vi "FieldAngleCalculation.vi"(8 "Previous Field Angle (rad)":sgl, 9 "Flux density magnitude (T)":sgl, 11 "Omega (rad/s)":sgl) -> (1 "New Field Angle (rad)":sgl, 2 "Bv (T)":sgl, 3 "Bu (T)":sgl)   [LabVIEW 2017]
uses:
  <vilib>/rvi/FXPMathLib/FxpSinAndCos/subVIs/nifxpmath_SinAndCos_SimConfig.ctl
  <vilib>/rvi/FXPMathLib/FxpSinAndCos/simVIs/DllFxpSinAndCosTemp_sub.vi
  <vilib>/rvi/FXPMathLib/FxpSinAndCos/XNode/nifxpmath_SinAndCos.xnode
panel:
  in  "Time Step (ms)":sgl=2.0
  # "Control parameters"
  # "Output"
  # "Inputs"
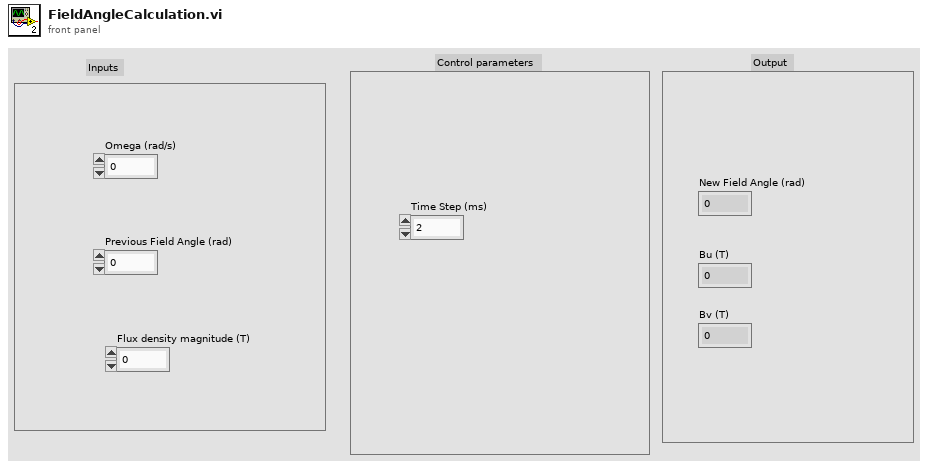
[diagram p1: front panel]
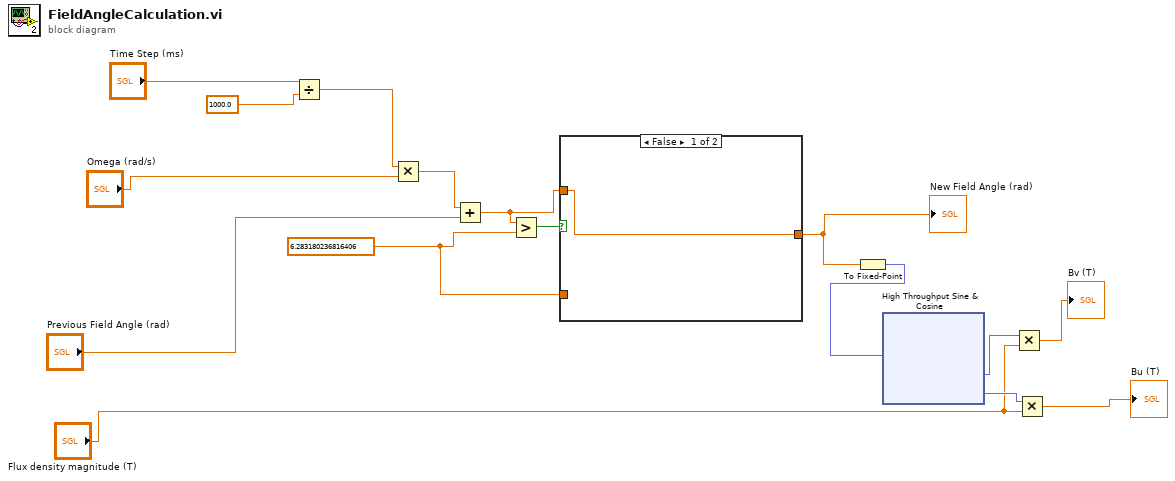
[diagram p0: block diagram]
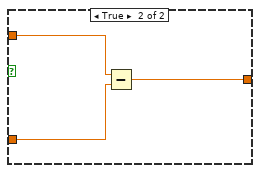
[diagram p2: hidden frame]
diagram:
  w8 = sgl 6.28318
  n1 = Divide(x="Time Step (ms)", y=sgl 1000.0) -> (x/y=w15:sgl)
  n2 = Multiply(x=w15, y="Omega (rad/s)") -> (x*y=w12:sgl)
  n3 = Add(x=w12, y="Previous Field Angle (rad)") -> (x+y=w9:sgl)
  n4 = Greater?(x=w9, y=w8) -> (0:w10:bool)
  n5 = case shown="False" w10 {
    tunnel: w9 -> [w17 w20]
    tunnel: w8 -> [_ w19]
    tunnel: [w17 w18] -> w7
    frame False {
    }
    frame True {
      n6 = Subtract(x=w20, y=w19) -> (x-y=w18:sgl)
    }
  }
  "New Field Angle (rad)" <- w7
  n7 = To Fixed-Point(number=w7) -> (fixed-point=w6:fxp<+/-,32,16>)  [unwired: 1 in]
  n8 = xnode "High Throughput Sine & Cosine"("x (pi)"=w6) -> ("sin(x)"=w2:fxp<+/-,16,2>, "cos(x)"=w5:fxp<+/-,16,2>)
  n9 = Multiply(x=w2, y="Flux density magnitude (T)") -> (x*y=→"Bv (T)":sgl)
  n10 = Multiply(x=w5, y="Flux density magnitude (T)") -> (x*y=→"Bu (T)":sgl)
